vi "ChekOF.vi"(8 "errin":errorcluster, 11 "OF in":string) -> (0 "errout":errorcluster, 1 "SN":string, 2 "version":string, 3 "PN":string, 4 "Réponse":string, 5 "ArrsurErr":bool)   [LabVIEW 2020]
doc: "Parse l'OF scané et verifie la forme"
uses:
  <vilib>/regexp/Match Regular Expression.xnode
panel:
  out "toute l'expression":string
  # "00078336_C|1|PCS||091937|"
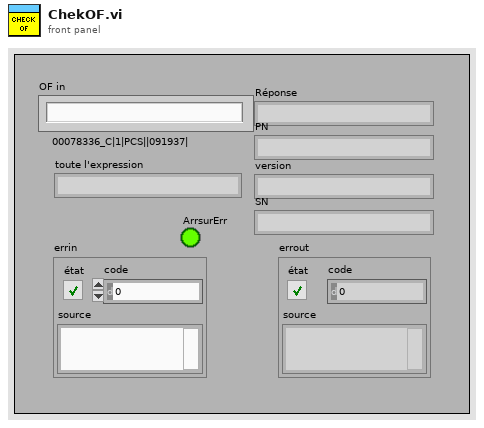
[diagram p1: front panel]
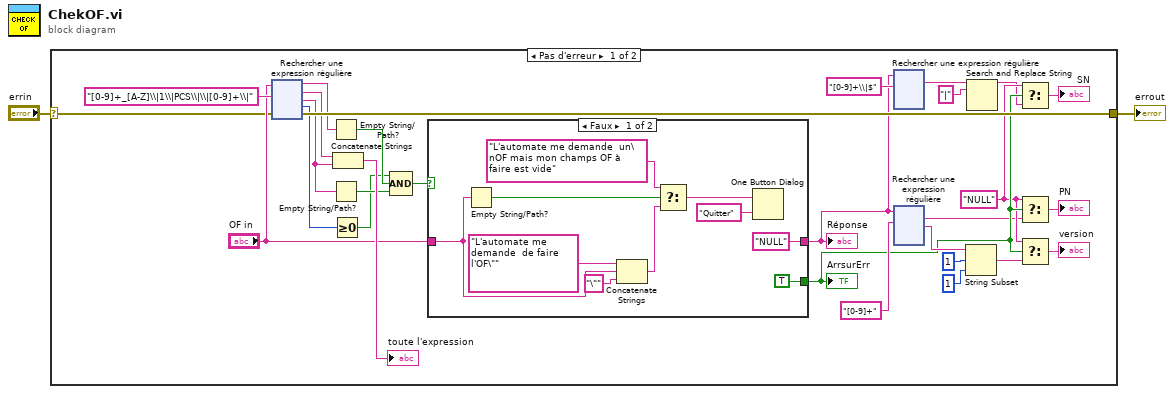
[diagram p0: block diagram]
diagram:
  n1 = case shown="Pas d'erreur" "errin" {
    selector: "errin" -> [w9 w385]
    tunnel: [w24 w385] -> w2
    frame No Error {
      w16 = "NULL"
      n2 = xnode "Rechercher une expression régulière"("chaîne en entrée"="OF in", "expression régulière"="[0-9]+_[A-Z]\\|1\\|PCS\\|\\|[0-9]+\\|", "entrée d'erreur"=w9) -> ("avant la correspondance"=w8:string, "toute l'expression"=w22:string, "après la correspondance"=w7:string, "offset après correspondance"=w23:i32, "sortie d'erreur"=w24:errorcluster)  [unwired: 3 in]
      n3 = Empty String/Path?(string/path=w8) -> (empty?=w6:bool)
      n4 = Empty String/Path?(string/path=w7) -> (empty?=w5:bool)
      n5 = Greater Or Equal To 0?(x=w23) -> (x >= 0?=w4:bool)
      n6 = Concatenate Strings(w22, w7) -> (→"toute l'expression":string)
      n7 = Compound Arithmetic op=AND ("Opérateur arithmétique")(w4, w6, w5) -> (w3:bool)
      n8 = case shown="Faux" w3 {
        tunnel: [TRUE _] -> w17
        tunnel: "OF in" -> [w150 w156]
        tunnel: ["NULL" ("OF in") w156] -> w18
        frame False {
          n9 = Empty String/Path?(string/path=w150) -> (empty?=w149:bool)
          n10 = Concatenate Strings("L'automate me demande  de faire l'OF\"" ("message"), w150, "\"" ("chaîne")) -> (w147:string)
          n11 = Select(t="L'automate me demande  un\nOF mais mon champs OF à faire est vide" ("message"), s=w149, f=w147) -> (s? t:f=w146:string)
          n12 = One Button Dialog(message=w146, button name ("OK")="Quitter" ("Nom du bouton F (\"Annuler\")")) -> ()  [unwired: 1 out]
        }
        frame True {
        }
      }
      "Réponse" <- w18
      "ArrsurErr" <- w17
      n13 = xnode "Rechercher une expression régulière"("chaîne en entrée"=w18, "expression régulière"="[0-9]+\\|$" ("chaîne en entrée")) -> ("toute l'expression"=w26:string)  [unwired: 4 in, 4 out]
      n14 = xnode "Rechercher une expression régulière"("chaîne en entrée"=w18, "expression régulière"="[0-9]+" ("chaîne en entrée")) -> ("toute l'expression"=w13:string, "après la correspondance"=w30:string)  [unwired: 4 in, 3 out]
      n15 = String Subset(string=w30, offset (0)=1, length (rest)=1 ("longueur (reste)")) -> (substring=w14:string)
      n16 = Search and Replace String(input string=w26, search string="|" ("chaîne recherchée")) -> (result string=w10:string)  [unwired: 6 in, 3 out]
      n17 = Select(t=w16, s=w17, f=w10) -> (s? t:f=→"SN":string)
      n18 = Select(t=w16, s=w17, f=w13) -> (s? t:f=→"PN":string)
      n19 = Select(t=w16, s=w17, f=w14) -> (s? t:f=→"version":string)
    }
    frame Error {
    }
  }
  "errout" <- w2
